vi "GetWindows.vi"(8 "No Error":errorcluster) -> (0 "Error Out":errorcluster, 3 "Windows [SDL_Window *]":T1[](array[typedef]) format="%.0x")   [LabVIEW 2026, in "SDL3.lvlib" / "Video.lvlib"]
doc: "<B>Summary</B>\nGet a list of valid windows."
uses:
  Video.lvlib
  <vilib>/Utility/error.llb/Error Cluster From Error Code.vi
  Stdinc/Stdinc.lvlib
  Error/Error.lvlib
  Lib/SDL3.dll
  SDL_Window--pointer.ctl
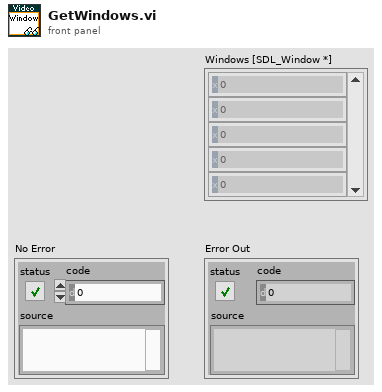
[diagram p1: front panel]
types:
  T1 = typedef "SDL3.lvlib/Video.lvlib/SDL_Window--pointer.ctl" = i64
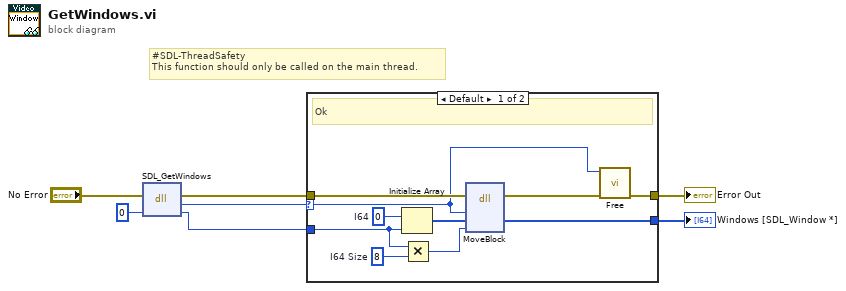
[diagram p0: block diagram]
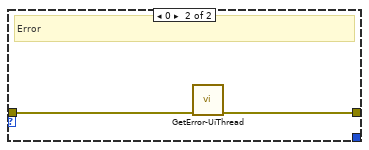
[diagram p2: hidden frame]
diagram:
  # "#SDL-ThreadSafety\nThis function should only be called on the main thread."
  n1 = dll-call lib="C:/Users/saukko/Dev/LV-SDL3/Sources/SDL3/Lib/SDL3.*" fn="SDL_GetWindows"(error in="No Error", "count"=0) -> (error out=w4:errorcluster, "return type"=w3:i64, "count"=w2:i32)  [unwired: 2 in, 1 out]
  n2 = case shown="Default" w3 {
    selector: w3 -> [w8 _]
    tunnel: w4 -> [w17 w19]
    tunnel: [w9 w18] -> w6
    tunnel: w2 -> [w14 _]
    tunnel: [w15 _] -> w1
    frame Default {
      w10 = i64 0  # I64
      w12 = 8  # I64 Size
      # "Ok"
      n3 = Initialize Array(w10, w14) -> (w16:i64[])
      n4 = Multiply(x=w14, y=w12) -> (x*y=w13:i32)
      n5 = dll-call lib="LabVIEW" fn="MoveBlock"(error in=w17, "Address"=w8, "Destination"=w16, "Size"=w13) -> (error out=w11:errorcluster, "Destination"=w15:i64[])  [unwired: 5 in, 1 out]
      n6 = call "Free.vi"("No Error"=w11, "Mem [void *]"=w8) -> ("Error Out"=w9:errorcluster)  [unwired: 9 in]
    }
    frame 0 {
      # "Error"
      n7 = call "GetError-UiThread.vi"("No Error"=w19) -> ("error out"=w18:errorcluster)  [unwired: 10 in]
    }
  }
  "Error Out" <- w6
  "Windows [SDL_Window *]" <- w1
